vi "Keysight E36300 Series Output List Sequence.vi"() -> ()   [LabVIEW 2020]
doc: "This example shows how to configure the source output sequence.\n\n<b>Notes:</b>\n(1)This VI is only available on the E36312A and E36313A models.\n(2)The list is up to 100 steps.\n(3)This VI overwrites previously programmed list."
uses:
  Keysight E36300 Series.lvlib
panel:
  in  "Step Value List (0.001)":dbl[](array[numeric]) format="%#_3g"
  in  "Time Point (0.01 sec)":dbl[](array[numeric])=[0.1] format="%#_3g"
  in  "End Trigger Signal List Step (F: Disable)":bool[](array[boolean])=[FALSE]
  in  "Begin Trigger Signal List Step (F: Disable)":bool[](array[boolean])=[FALSE]
  in  "Termination Value (0: Before List Starting Value)":i32(ring) items=["Before List Starting Value", "Last Step Value"]
  in  "Enable List Continuously (F: Disable)":bool
  in  "Stop Output":bool
  out "Actual Level (V)":dbl[](array[numeric]) format="%.2g"
  in  "Channel (1)":string="1"
  in  "Execution Times (5)":i32=5
  in  "List Step Setting (0: Automatically)":i32(ring) items=["Automatically", "Once"]
  in  "List (0: Current List)":i32(ring) items=["Current List", "Voltage List"]
  in  "VISA resource name":refnum<visa-resource-name>
  # "(c) 2019 - 2021 National Instruments.  ALL RIGHTS RESERVED."
  # "This VI is only available on the E36312A and E36313A models."
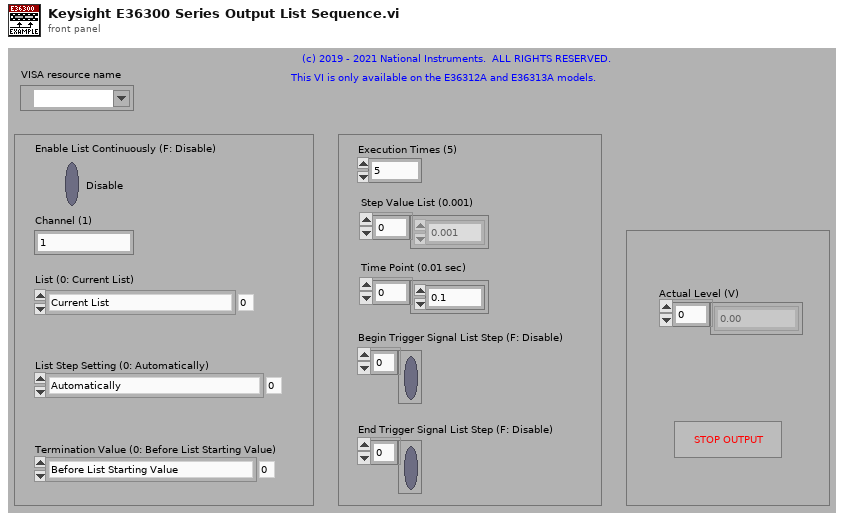
[diagram p1: front panel]
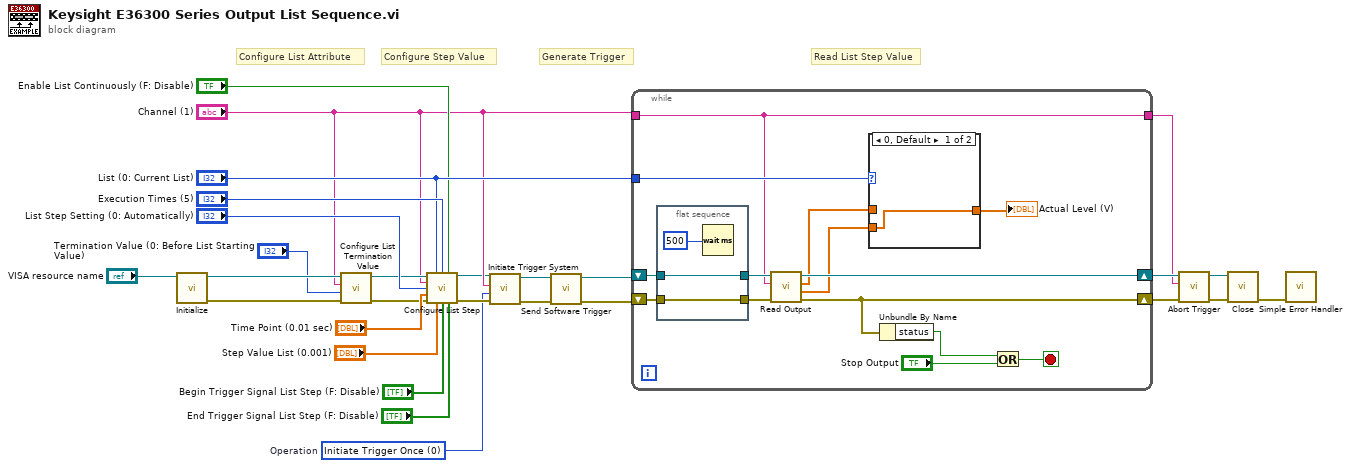
[diagram p0: block diagram]
diagram:
  w4 = u16 0 items=["Initiate Trigger Once", "Initiate Trigger Continuously", "Stop Continuously Trigger"]  # Operation
  # "Generate Trigger"
  # "Read List Step Value"
  # "Configure Step Value"
  # "Configure List Attribute"
  n1 = call "Initialize.vi"("VISA resource name"="VISA resource name") -> ("error out"=w23:errorcluster, "VISA resource name out"=w24:refnum<visa-resource-name>)  [unwired: 9 in]
  n2 = call "Configure List Termination Value.vi"("error in (no error)"=w23, "Termination Value (0: Before List Starting Value)"="Termination Value (0: Before List Starting Value)", "Channel (1)"="Channel (1)", "VISA resource name"=w24) -> ("error out"=w10:errorcluster, "VISA resource name out"=w11:refnum<visa-resource-name>)  [unwired: 6 in]
  n3 = call "Configure List Step.vi"("VISA resource name"=w11, "List (0: Current List)"="List (0: Current List)", "Execution Times (1)"="Execution Times (5)", "Enable List Continuously (F: Disable)"="Enable List Continuously (F: Disable)", "Channel (1)"="Channel (1)", "List Step Setting (0: Automatically)"="List Step Setting (0: Automatically)", "Time Point (0 sec)"="Time Point (0.01 sec)", "error in (no error)"=w10, "Step Value List (0.001)"="Step Value List (0.001)", "Begin Trigger Signal List Step (F: Disable)"="Begin Trigger Signal List Step (F: Disable)", "End Trigger Signal List Step (F: Disable)"="End Trigger Signal List Step (F: Disable)") -> ("VISA resource name out"=w6:refnum<visa-resource-name>, "error out"=w5:errorcluster)  [unwired: 3 in]
  n4 = call "Initiate Trigger System.vi"("error in (no error)"=w5, "Operation (0 : Initiate Trigger Once)"=w4, "Channel (1)"="Channel (1)", "VISA resource name"=w6) -> ("error out"=w8:errorcluster, "VISA resource name out"=w9:refnum<visa-resource-name>)  [unwired: 6 in]
  n5 = call "Send Software Trigger.vi"("error in (no error)"=w8, "VISA resource name"=w9) -> ("error out"=w2:errorcluster, "VISA resource name out"=w3:refnum<visa-resource-name>)  [unwired: 8 in]
  n6 = while {
    tunnel: "Channel (1)" -> [w29]
    tunnel: "List (0: Current List)" -> [w39]
    shift-right: [w33] -> w15
    shift-left: w2 -> [w36]
    shift-right: [w42] -> w16
    shift-left: w3 -> [w37]
    tunnel: [w29] -> w12
    stop <- w30 stop-if-true
    n7 = flat-sequence {
      tunnel: w37 -> [w44]
      tunnel: w36 -> [w43]
      tunnel: [w44] -> w35
      tunnel: [w43] -> w34
      frame #0 {
        n8 = Wait (ms)(milliseconds to wait=500) -> ()  [unwired: 1 out]
      }
    }
    n9 = call "Read Output.vi"("error in (no error)"=w34, "Channel (1)"=w29, "VISA resource name"=w35) -> ("error out"=w33:errorcluster, "Actual Current Level (A)"=w40:dbl[], "Actual Voltage Level (V)"=w41:dbl[], "VISA resource name out"=w42:refnum<visa-resource-name>)  [unwired: 5 in]
    n10 = case shown="0, Default" w39 {
      tunnel: w41 -> [_ w47]
      tunnel: w40 -> [w46 _]
      tunnel: [w46 w47] -> w38
      frame 0, Default {
      }
      frame 1 {
      }
    }
    "Actual Level (V)" <- w38
    n11 = Unbundle By Name(w33) -> ("status"=w32:bool)
    n12 = Or(x=w32, y="Stop Output") -> (x .or. y?=w30:bool)
  }
  n13 = call "Abort Trigger.vi"("error in (no error)"=w15, "Channel (1)"=w12, "VISA resource name"=w16) -> ("error out"=w13:errorcluster, "VISA resource name out"=w14:refnum<visa-resource-name>)  [unwired: 7 in]
  n14 = call "Close.vi"("error in (no error)"=w13, "VISA resource name"=w14) -> ("error out"=w27:errorcluster)  [unwired: 9 in]
  n15 = call <vilib>:"Simple Error Handler.vi"("error in (no error)"=w27) -> ()  [unwired: 4 in, 5 out]
